vi "screen for automatic display mode.vi"() -> ()   [LabVIEW 2022 SP3]
panel:
  in  "?":dbl(slide) scale=0.0..10.0
  in  "?":dbl(slide) scale=0.0..10.0
  out "?":dbl format="%#.6f"
  out "?":dbl format="%#.6f"
  out "?":dbl format="%#.6f"
  out "?":dbl format="%#.6f"
  out "?":bool
  out "?":string="Job name Line 1 Line 2"
  out "?":timestamp format="%<%d %b %Y | %H:%M>T"
  out "?":timestamp format="%<%-%Hh %Mm %Ss>T"
  in  "?":bool
  out "?":picture
  out "?":picture
  # "Procedures completed"
  # "/"
  # "/"
  # "JOB STARTED ON"
  # "Remaining"
  # "Y Axis"
  # "X Axis"
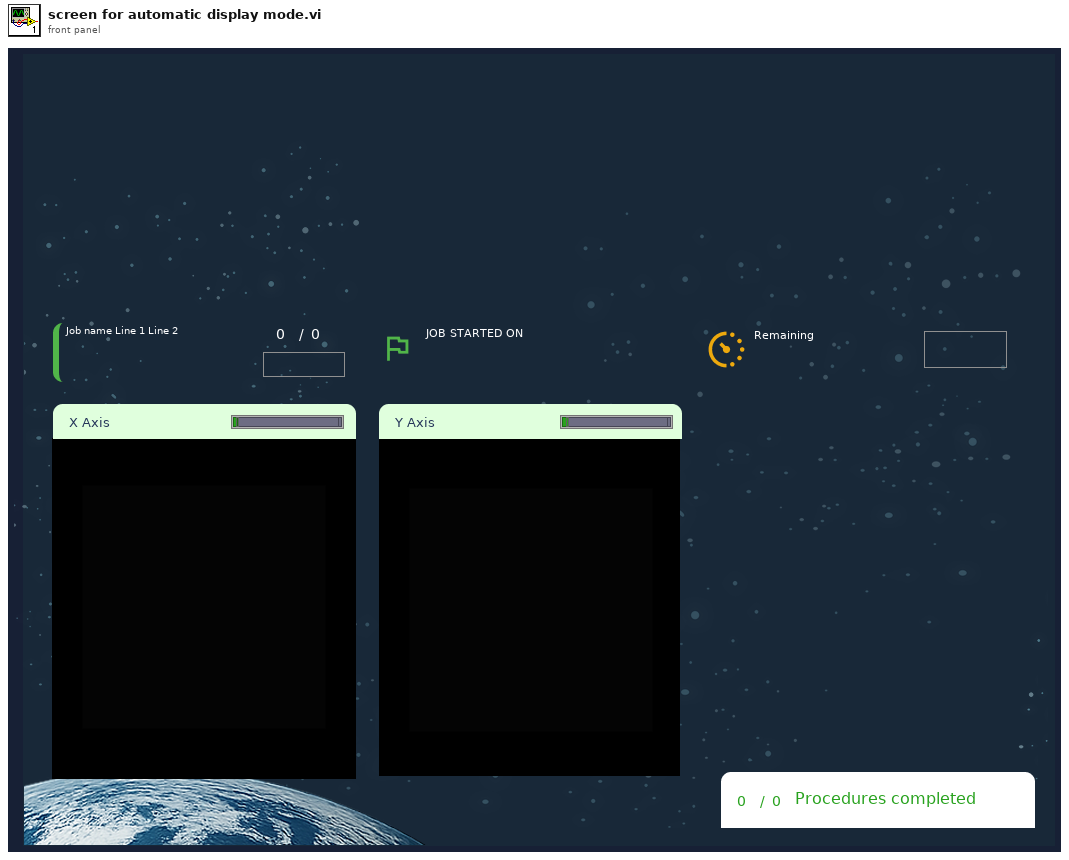
[diagram p1: front panel]
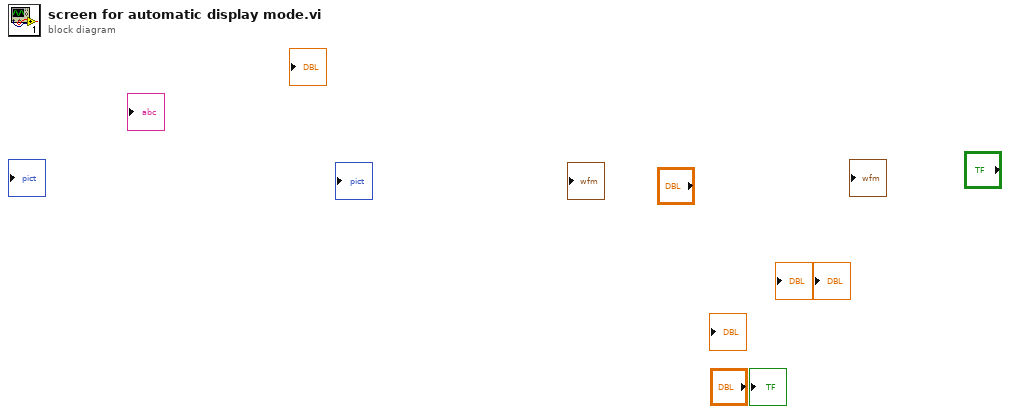
[diagram p0: block diagram]
diagram:
